vi "getScriptoObjFromClassName.vi"(8 "error in (no error)":errorcluster, 11 "className":string) -> (0 "error out":errorcluster, 2 "found?":bool, 3 "Generic":refnum<class "Generic.lvclass">)   [LabVIEW 2023, in "TLC_Scripto.lvlib"]
uses:
  TLC_Scripto.lvlib
  Generic/Generic.lvclass
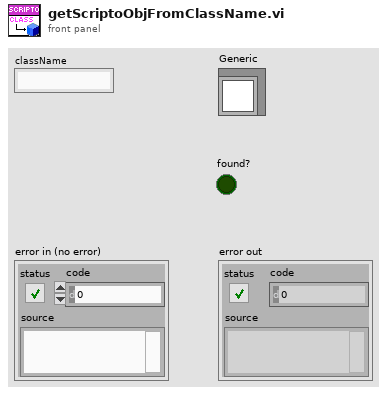
[diagram p1: front panel]
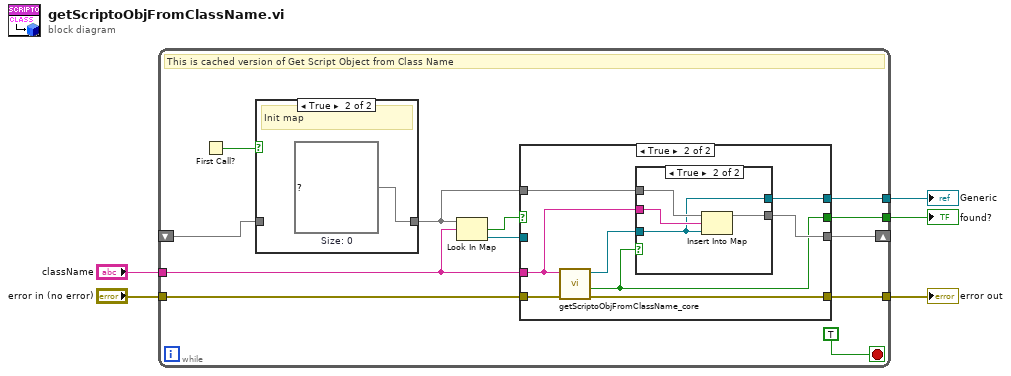
[diagram p0: block diagram]
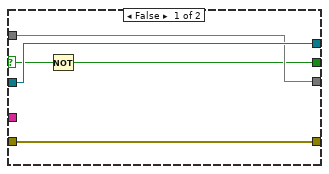
[diagram p3: hidden frame]
diagram:
  n1 = while {
    tunnel: "className" -> [w15]
    tunnel: "error in (no error)" -> [w17]
    tunnel: [w12] -> w3
    shift-right: [w11] -> _
    shift-left: _ -> [w8]
    tunnel: [w7] -> w2
    tunnel: [w6] -> w1
    stop <- TRUE stop-if-true
    # "This is cached version of Get Script Object from Class Name"
    n2 = First Call?() -> (First Call?: T/F=w10:bool)
    n3 = case shown="True" w10 {
      tunnel: [w18 w19] -> w9
      tunnel: w8 -> [w18 _]
      frame False {
      }
      frame True {
        w19 = map{string, refnum<class "Generic.lvclass">} {}  # Size: 0
        # "Init map"
      }
    }
    n4 = Look In Map(map=w9, key=w15) -> (key not found?=w14:bool, value=w13:refnum<class "Generic.lvclass">)  [unwired: 1 in]
    n5 = case shown="True" w14 {
      selector: w14 -> [w21 _]
      tunnel: w15 -> [_ w29]
      tunnel: w17 -> [w22 w30]
      tunnel: w13 -> [w24 _]
      tunnel: [w24 w26] -> w12
      tunnel: w9 -> [w23 w32]
      tunnel: [w23 w31] -> w11
      tunnel: [w22 w25] -> w7
      tunnel: [w20 w28] -> w6
      frame False {
        n6 = Not(x=w21) -> (.not. x?=w20:bool)
      }
      frame True {
        n7 = call "getScriptoObjFromClassName_core.vi"("error in (no error)"=w30, "className"=w29) -> ("error out"=w25:errorcluster, "found?"=w28:bool, "matchingObj"=w27:refnum<class "Generic.lvclass">)  [unwired: 7 in]
        n8 = case shown="True" w28 {
          tunnel: w32 -> [w33 w37]
          tunnel: [w33 w36] -> w31
          tunnel: w29 -> [_ w35]
          tunnel: w27 -> [_ w34]
          tunnel: [_ w34] -> w26
          frame False {
          }
          frame True {
            n9 = Insert Into Map(map in=w37, key=w35, value=w34) -> (map out=w36:map{string, refnum<class "Generic.lvclass">})  [unwired: 2 out]
          }
        }
      }
    }
  }
  "Generic" <- w3
  "error out" <- w2
  "found?" <- w1
